vi "ABR3-Init Stim Chans (develop).vi"(0 "Stimulus":T29={"Ear"=enum."Left", "Waveform"=enum."TONE PIP", "Frequency (kHz)"="", "Rep rate (/sec)"=30.0, "Alternate Polarity"=FALSE, "WavFiles"="", "Level (dB SPL)"=30.0, "WavFolder"=path "", "Chirp"={"Type"=enum."AN latency-corrected", "Duration (ms)"=0.0, "Fmin (kHz)"=0.0, "Fmax (kHz)"=0.0, "precompensate"=FALSE}, "Noise"={"Seed"=0, "InvFilt"=FALSE, "AWeight"=FALSE, "afile"=path "", "Filter"={"Type"=enum."Lowpass", "CF (kHz)"=0.0, "BW (kHz)"=0.0, "Cascade"=FALSE, "Quadrature"=FALSE, "Scale Factor"=0.0, "Stages"=[], "Class"=enum."Elliptic", "Order"=0, "BWUnits"=enum."Linear"}}}, 1 "Masker":T27, 2 "Data Folder":path, 9 "Hidden":T28={"AI Samp Rate Hz"=25000.0, "AO Samp Rate Hz"=100000.0, "Duration (ms)"=5.0, "Ramp (ms)"=0.5, "Click width (us)"=0.0, "ITI"=enum."Rate"}, 11 "error in (no error)":errorcluster) -> (4 "StimChans":T4[](xcontrol), 15 "error out":errorcluster)   [LabVIEW 2020]
uses:
  TypeDefs/ABR3-Stimulus.ctl
  Utility VIs/Type Defs/Left-Right ring.ctl
  TypeDefs/ABR-Waveform Enum.ctl
  Signal Synthesis VIs/Controls/Advanced Filter XCtl/Advanced Filter XCtl.xctl
  TypeDefs/ABR-Hidden Params.ctl
  TypeDefs/ABR3-Masker Spec.ctl
  Signal Synthesis VIs/Controls/Level XCtl/Level XCtl.xctl
  Signal Synthesis VIs/Controls/Stimulus Channel (Full)/Stimulus Channel (Full).xctl
  Signal Synthesis VIs/Controls/Multichannel (Full)/Multichannel (Full).xctl
  Signal Synthesis VIs/Waveform VIs/Pulse Train VIs/Pulse Train Params.ctl
  Signal Synthesis VIs/Waveform VIs/Pulse Train VIs/Pulse Polarity.ctl
  Signal Synthesis VIs/Waveform VIs/Pulse Train VIs/PT-Continuous State.ctl
  Signal Synthesis VIs/Controls/Level XCtl/Level Units.ctl
  Signal Synthesis VIs/Controls/Waveform XCtl/Waveform Enum.ctl
  Utility VIs/Type Defs/Speaker ring.ctl
panel:
  in  "Pulse Train Params":T1
  in  "Dummy":T26(xcontrol)
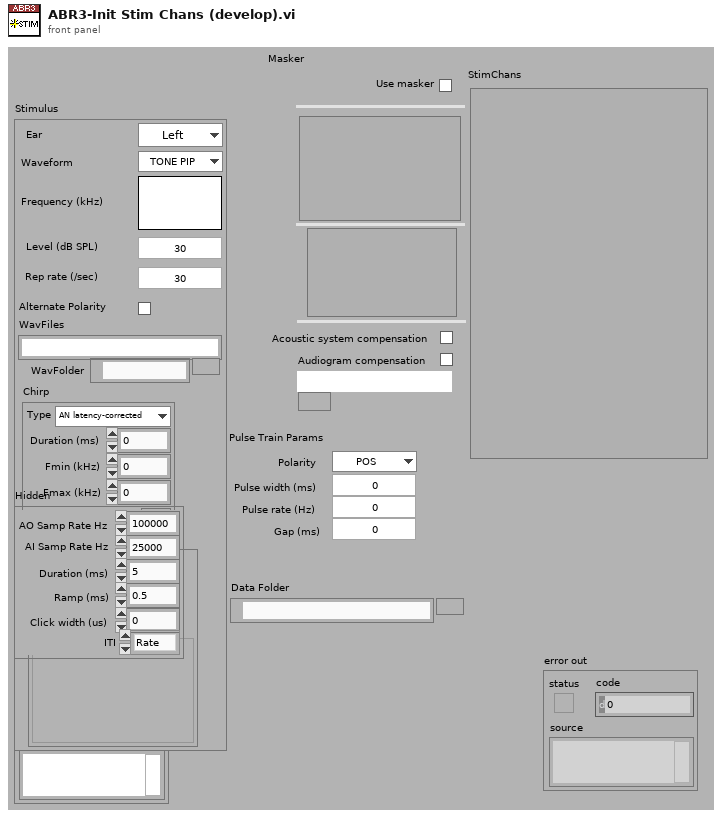
[diagram p1: front panel]
types:
  T1 = typedef "Pulse Train Params.ctl" = cluster{"Pulse width (us)":dbl, "Pulse rate (Hz)":dbl, "Gap (ms)":dbl, "Polarity":T2, "PT State":T3, "Asynch":bool}
  T2 = typedef "Pulse Polarity.ctl" = enum16{"POS", "NEG", "POS-NEG", "NEG-POS"}
  T3 = typedef "PT-Continuous State.ctl" = cluster{"Template":dbl[], "Nperiod":i32, "Index":i32, "Pulse Rate (Hz)":dbl, "Phase (cycles)":dbl, "Noff":i32}
  T4 = typedef "Stimulus Channel (Full).xctl/Full Stimulus Channel Data.ctl" = cluster{"Waveform":T5, "Filter":T19, "Burst":T21, "Level":T22, "Name":string, "Advanced":T24, "SAM":T25}
  T5 = typedef "Waveform XCtl.xctl/Waveform Data.ctl" = cluster{"Type":T6, "Tone":T7, "Pulse Train":T1, "Noise":T8, "File":T9, "FMSweep":T10, "Chirp Train":T11, "Complex Tone":cluster{"Params":T13, "Data":T15}, "Moving Ripple":T16}
  T6 = typedef "Waveform Enum.ctl" = enum16{"OFF", "Tone", "Noise", "Pulse Train", "File", "FM Sweep", "Chirp Train", "Complex Tone", "FM Tone", "Moving Ripple"}
  T7 = typedef "Tone Params.ctl" = cluster{"Frequency (kHz)":dbl, "Last Freq":dbl, "Last Phase":dbl}
  T8 = typedef "Noise Params.ctl" = cluster{"InvFilt":bool, "Noise":dbl[], "CurPt":i32, "Aweight":bool, "Seed":i32, "afile":path}
  T9 = typedef "StimFile-Params.ctl" = cluster{"Filename":path, "Signal":dbl[], "Channel":i32, "stream":bool, "offset":i32, "nreps":i32, "loops":i32, "Tokens":i32, "Randomize":bool, "order":i32[]}
  T10 = typedef "FM Sweep Params.ctl" = cluster{"Rate (oct/s)":dbl, "Fmin (Hz)":dbl, "Fmax (Hz)":dbl, "Ramp (ms)":dbl, "Linear":bool}
  T11 = typedef "Chirp Train.ctl" = cluster{"Params":T12, "Data":cluster{"WF":dbl[]}}
  T12 = typedef "Chirp Train Params.ctl" = cluster{"Fmin (kHz)":dbl, "Fmax (kHz)":dbl, "Compensate":bool, "Duration (ms)":dbl}
  T13 = typedef "CT-Params.ctl" = cluster{"F0 (Hz)":dbl, "Band":cluster{"Flow (Hz)":dbl, "Fhigh (Hz)":dbl}, "Phase":T14, "Min F0 (Hz)":dbl, "Max F0 (Hz)":dbl, "ContinRandPhase":bool, "Max peak factor":dbl, "Max mod depth":dbl, "MinHarmNum":i32, "MaxHarmNum":i32, "Level Mode":enum16{"per component", "overall rms"}, "% jitter":dbl}
  T14 = typedef "CT-Phase Enum.ctl" = enum16{"Cosine", "Random", "Alternating"}
  T15 = typedef "CT-Runtime Data.ctl" = cluster{"Ncomp":i32, "MinHarm":i32, "Phase":dbl[], "Amplitude":dbl[], "Npts/frame":i32, "Last F0":dbl, "Fmin":dbl, "Fmax":dbl, "Lslope":dbl, "randphase":bool, "overall rms":bool, "fmult":dbl[], "jittered":bool}
  T16 = typedef "Moving Ripple.ctl" = cluster{"Params":T17, "Data":T18}
  T17 = typedef "Moving Ripple.Params.ctl" = cluster{"Fmin":dbl, "Fmax":dbl, "Density":dbl, "Velocity":dbl, "Depth":dbl, "Phase":dbl, "Comp/oct":i32}
  T18 = typedef "Moving Ripple.Data.ctl" = cluster{"Freq":dbl[], "A":dbl[], "phase":dbl[], "Phase":dbl}
  T19 = typedef "Advanced Filter XCtl.xctl/Filter Data.ctl" = cluster{"Type":enum16{"Lowpass", "Highpass", "Bandpass", "Bandstop", "OFF"}, "CF (kHz)":dbl, "BW (kHz)":dbl, "Cascade":bool, "Quadrature":bool, "Scale Factor":dbl, "Stages":cluster{"IIR Filter":cluster{"filter structure":enum32{"IIR 2nd Order", "IIR 4th Order"}, "Reverse Coefficients":dbl[], "Forward Coefficients":dbl[]}, "State":dbl[]}[], "Class":enum16{"Elliptic", "Butterworth"}, "Order":i32, "BWUnits":T20}
  T20 = typedef "Filter-Bandwidth Units.ctl" = enum16{"Linear", "Octaves", "Min-Max"}
  T21 = typedef "Burst Control.xctl/Burst Data.ctl" = cluster{"Active":bool, "Delay (ms)":dbl, "Duration (ms)":dbl, "Ramp (ms)":dbl, "Rate (Hz)":dbl, "Trepeat (ms)":dbl, "Repeat":bool}
  T22 = typedef "Level XCtl.xctl/Level Data.ctl" = cluster{"Level":dbl, "Units":T23, "Max":dbl, "Multiplier":dbl, "Cal File":path, "Cal":cluster{"Freq (Hz)":dbl[], "Mag (dB SPL)":dbl[], "Phase (deg)":dbl[]}}
  T23 = typedef "Level Units.ctl" = enum16{"dB atten", "dB SPL", "dB re 1 Vrms", "dB V/Hz½", "mW", "dB HL", "Volts", "dB mW"}
  T24 = typedef "Advanced Stimulus Options.xctl/Advanced Stimulus Options.ctl" = cluster{"Rep Mask":string, "AltPol":bool, "Var":string, "Expr":string, "Persist":bool}
  T25 = typedef "SAM Params.ctl" = cluster{"Active":bool, "Frequency (Hz)":dbl, "Depth":dbl, "Init Phase (cycles)":dbl, "phase (degrees)":dbl, "Asynch":bool}
  T26 = cluster{"Waveform":T5, "Filter":T19, "Burst":T21, "Level":T22, "Name":string, "Advanced":T24, "SAM":T25}
  T27 = typedef "ABR3-Masker Spec.ctl" = cluster{"Filter":cluster{"Type":enum16{"Lowpass", "Highpass", "Bandpass", "Bandstop", "OFF"}, "CF (kHz)":dbl, "BW (kHz)":dbl, "Cascade":bool, "Quadrature":bool, "Scale Factor":dbl, "Stages":cluster{"IIR Filter":cluster{"filter structure":enum32{"IIR 2nd Order", "IIR 4th Order"}, "Reverse Coefficients":dbl[], "Forward Coefficients":dbl[]}, "State":dbl[]}[], "Class":enum16{"Elliptic", "Butterworth"}, "Order":i32, "BWUnits":T20}, "Use masker":bool, "Level":cluster{"Level":dbl, "Units":T23, "Max":dbl, "Multiplier":dbl, "Cal File":path, "Cal":cluster{"Freq (Hz)":dbl[], "Mag (dB SPL)":dbl[], "Phase (deg)":dbl[]}}, "Audiogram Comp":bool, "Audiogram File":path, "InvFilt":bool}
  T28 = typedef "ABR-Hidden Params.ctl" = cluster{"AI Samp Rate Hz":dbl, "AO Samp Rate Hz":dbl, "Duration (ms)":dbl, "Ramp (ms)":dbl, "Click width (us)":dbl, "ITI":enum16{"Rate", "Interval"}}
  T29 = typedef "ABR3-Stimulus.ctl" = cluster{"Ear":T30, "Waveform":T31, "Frequency (kHz)":string, "Rep rate (/sec)":dbl, "Alternate Polarity":bool, "WavFiles":string, "Level (dB SPL)":dbl, "WavFolder":path, "Chirp":cluster{"Type":enum16{"AN latency-corrected", "Arbitrary"}, "Duration (ms)":dbl, "Fmin (kHz)":dbl, "Fmax (kHz)":dbl, "precompensate":bool}, "Noise":cluster{"Seed":i32, "InvFilt":bool, "AWeight":bool, "afile":path, "Filter":cluster{"Type":enum16{"Lowpass", "Highpass", "Bandpass", "Bandstop", "OFF"}, "CF (kHz)":dbl, "BW (kHz)":dbl, "Cascade":bool, "Quadrature":bool, "Scale Factor":dbl, "Stages":cluster{"IIR Filter":cluster{"filter structure":enum32{"IIR 2nd Order", "IIR 4th Order"}, "Reverse Coefficients":dbl[], "Forward Coefficients":dbl[]}, "State":dbl[]}[], "Class":enum16{"Elliptic", "Butterworth"}, "Order":i32, "BWUnits":T20}}}
  T30 = typedef "Left-Right ring.ctl" = enum16{"Right", "Left"}
  T31 = typedef "ABR-Waveform Enum.ctl" = enum16{"TONE PIP", "CLICK", "FILE", "CHIRP", "NOISE", "VERHULST"}
  T32 = enum16{"Lowpass", "Highpass", "Bandpass", "Bandstop", "OFF"}
  T33 = typedef "Speaker ring.ctl" = enum16{"Right primary", "Right secondary", "Left primary", "Left secondary"}
  T34 = cluster{"Type":enum16{"Lowpass", "Highpass", "Bandpass", "Bandstop", "OFF"}, "CF (kHz)":dbl, "BW (kHz)":dbl, "Cascade":bool, "Quadrature":bool, "Scale Factor":dbl, "Stages":cluster{"IIR Filter":cluster{"filter structure":enum32{"IIR 2nd Order", "IIR 4th Order"}, "Reverse Coefficients":dbl[], "Forward Coefficients":dbl[]}, "State":dbl[]}[], "Class":enum16{"Elliptic", "Butterworth"}, "Order":i32, "BWUnits":T20}
  T35 = cluster{"Level":dbl, "Units":T23, "Max":dbl, "Multiplier":dbl, "Cal File":path, "Cal":cluster{"Freq (Hz)":dbl[], "Mag (dB SPL)":dbl[], "Phase (deg)":dbl[]}}
  T36 = cluster{"Waveform":T5, "Filter":T19, "Burst":T21, "Level":T22, "Name":string, "Advanced":T24, "SAM":T25}[]
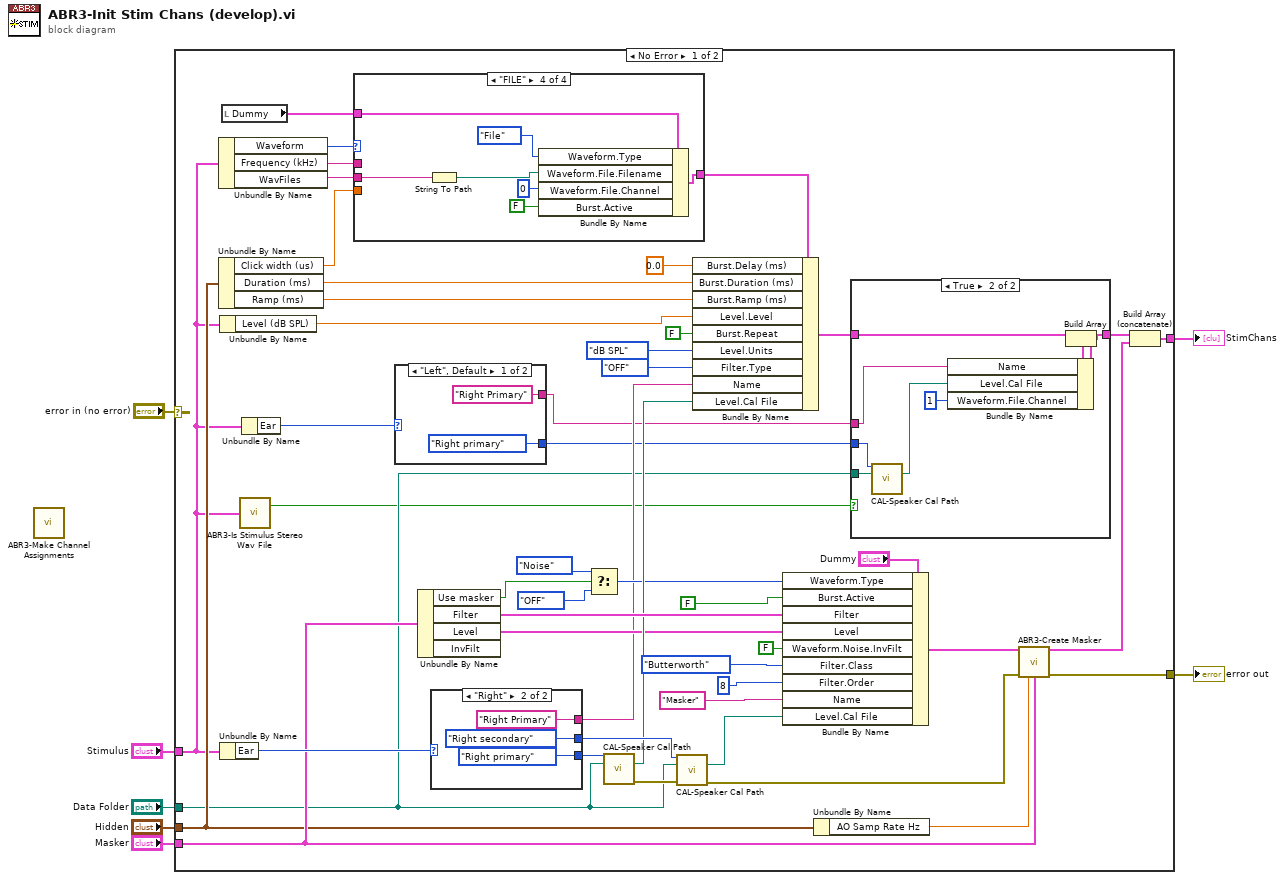
[diagram p0: block diagram]
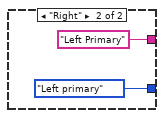
[diagram p2: hidden frame]
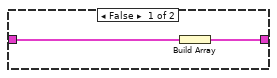
[diagram p3: hidden frame]
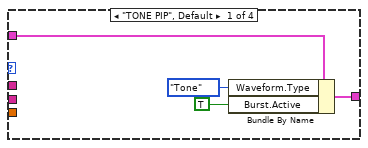
[diagram p4: hidden frame]
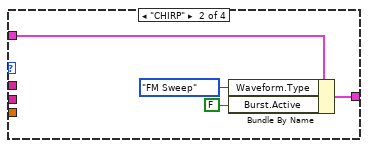
[diagram p5: hidden frame]
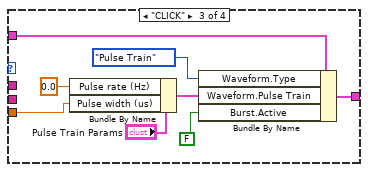
[diagram p6: hidden frame]
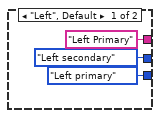
[diagram p7: hidden frame]
diagram:
  n1 = call "ABR3-Make Channel Assignments.vi"() -> ()  [unwired: 12 in, 4 out]
  n2 = case shown="No Error" "error in (no error)" {
    selector: "error in (no error)" -> [_ w99]
    tunnel: "Hidden" -> [w19 _]
    tunnel: [w46 _] -> w6
    tunnel: "Stimulus" -> [w9 _]
    tunnel: "Data Folder" -> [w13 _]
    tunnel: [w22 w99] -> w2
    tunnel: "Masker" -> [w20 _]
    frame No Error {
      n3 = Unbundle By Name(w9) -> ("Waveform"=w33:T31, "Frequency (kHz)"=w32:string, "WavFiles"=w31:string)
      n4 = Unbundle By Name(w19) -> ("Click width (us)"=w35:dbl, "Duration (ms)"=w54:dbl, "Ramp (ms)"=w53:dbl)
      n5 = Unbundle By Name(w9) -> ("Level (dB SPL)"=w24:dbl)
      n6 = Unbundle By Name(w9) -> ("Ear"=w42:T30)
      n7 = local read "Dummy"() -> (w36:T26)
      n8 = call "ABR3-Is Stimulus Stereo Wav File.vi"("Stimulus"=w9) -> ("Is Stereo Wav File"=w8:bool)  [unwired: 1 out]
      n9 = Unbundle By Name(w9) -> ("Ear"=w12:T30)
      n10 = case shown="\"FILE\"" w33 {
        tunnel: w36 -> [w73 w77 w83 w92]
        tunnel: w35 -> [_ _ w80 _]
        tunnel: [w72 w76 w79 w90] -> w34
        tunnel: w32 -> [_ _ _ _]
        tunnel: w31 -> [_ _ _ w88]
        frame "TONE PIP", Default {
          n11 = Bundle By Name(cluster=w73, "Waveform.Type"=Waveform_Enum."Tone", "Burst.Active"=TRUE) -> (w72:T26)
        }
        frame "CHIRP" {
          n12 = Bundle By Name(cluster=w77, "Waveform.Type"=Waveform_Enum."FM Sweep", "Burst.Active"=FALSE) -> (w76:T26)
        }
        frame "CLICK" {
          n13 = Bundle By Name(cluster="Pulse Train Params", "Pulse rate (Hz)"=0.0, "Pulse width (us)"=w80) -> (w82:T1)
          n14 = Bundle By Name(cluster=w83, "Waveform.Type"=Waveform_Enum."Pulse Train", "Waveform.Pulse Train"=w82, "Burst.Active"=FALSE) -> (w79:T26)
        }
        frame "FILE" {
          n15 = String To Path(string=w88) -> (path=w87:path)
          n16 = Bundle By Name(cluster=w92, "Waveform.Type"=Waveform_Enum."File", "Waveform.File.Filename"=w87, "Waveform.File.Channel"=0, "Burst.Active"=FALSE) -> (w90:T26)
        }
      }
      n17 = case shown="\"Left\", Default" w12 {
        tunnel: [Speaker_ring."Right primary" ("Speaker") Speaker_ring."Left primary" ("Speaker")] -> w10
        tunnel: ["Right Primary" ("Name") "Left Primary" ("Name")] -> w11
        frame "Left", Default {
        }
        frame "Right" {
        }
      }
      n18 = Unbundle By Name(w20) -> ("Use masker"=w40:bool, "Filter"=w47:T34, "Level"=w28:T35)  [unwired: 1 out]
      n19 = case shown="\"Right\"" w42 {
        tunnel: [Speaker_ring."Left primary" ("Speaker") Speaker_ring."Right primary" ("Speaker")] -> w45
        tunnel: [Speaker_ring."Left secondary" ("Speaker") Speaker_ring."Right secondary" ("Speaker")] -> w44
        tunnel: ["Left Primary" ("Name") "Right Primary" ("Name")] -> w25
        frame "Left", Default {
        }
        frame "Right" {
        }
      }
      n20 = Select(t=Waveform_Enum."Noise", s=w40, f=Waveform_Enum."OFF" ("Waveform.Type")) -> (s? t:f=w38:T6)
      n21 = call "CAL-Speaker Cal Path.vi"("Speaker"=w45, "Data Folder"=w13) -> ("Cal Path"=w41:path, "error out"=w43:errorcluster)  [unwired: 12 in]
      n22 = call "CAL-Speaker Cal Path.vi"("Speaker"=w44, "Data Folder"=w13, "error in (no error)"=w43) -> ("Cal Path"=w27:path, "error out"=w23:errorcluster)  [unwired: 11 in]
      n23 = Bundle By Name(cluster=w34, "Burst.Delay (ms)"=0.0, "Burst.Duration (ms)"=w54, "Burst.Ramp (ms)"=w53, "Level.Level"=w24, "Burst.Repeat"=FALSE, "Level.Units"=Level_Units."dB SPL" ("Level.Mode"), "Filter.Type"=T32."OFF", "Name"=w25, "Level.Cal File"=w41) -> (w14:T26)
      n24 = Bundle By Name(cluster="Dummy", "Waveform.Type"=w38, "Burst.Active"=FALSE, "Filter"=w47, "Level"=w28, "Waveform.Noise.InvFilt"=FALSE, "Filter.Class"=enum16{"Elliptic", "Butterworth"}."Butterworth", "Filter.Order"=8, "Name"="Masker", "Level.Cal File"=w27) -> (w21:T26)
      n25 = Unbundle By Name(w19) -> ("AO Samp Rate Hz"=w18:dbl)
      n26 = case shown="True" w8 {
        tunnel: [w60 w69] -> w15
        tunnel: w14 -> [w61 w68]
        tunnel: w13 -> [_ w66]
        tunnel: w11 -> [_ w65]
        tunnel: w10 -> [_ w64]
        frame False {
          n27 = Build Array(w61) -> (w60:T36)
        }
        frame True {
          n28 = call "CAL-Speaker Cal Path.vi"("Speaker"=w64, "Data Folder"=w66) -> ("Cal Path"=w63:path)  [unwired: 12 in, 1 out]
          n29 = Bundle By Name(cluster=w68, "Name"=w65, "Level.Cal File"=w63, "Waveform.File.Channel"=1) -> (w67:T26)
          n30 = Build Array(w68, w67) -> (w69:T36)
        }
      }
      n31 = call "ABR3-Create Masker.vi"("StimChan"=w21, "error in (no error)"=w23, "Sampling rate (Hz)"=w18, "Masker"=w20) -> ("Stimulus Channel out"=w17:T4, "error out"=w22:errorcluster)  [unwired: 10 in]
      n32 = Build Array (concatenate)(w15, w17) -> (w46:T4[])
    }
    frame Error {
    }
  }
  "error out" <- w2
  "StimChans" <- w6
